vi "hse-configuration_ReadBooleanKey.vi"(8 "error in (no error)":errorcluster, 9 "Key":string, 10 "Section":string, 11 "hse-config-ini in":refnum<class "hse-config-ini.lvclass">) -> (0 "error out":errorcluster, 2 "Value":bool, 3 "hse-config-ini out":refnum<class "hse-config-ini.lvclass">)   [LabVIEW 2020, in "hse-config-ini.lvclass"]
doc: "Reads the numeric configuration value (I32) identified by <b>section</b> and <b>key</b> from the configuration object\n\n____\nHAMPEL SOFTWARE ENGINEERING v3.8.0 (2023-12-18 14:41)"
uses:
  hse-config-ini.lvclass
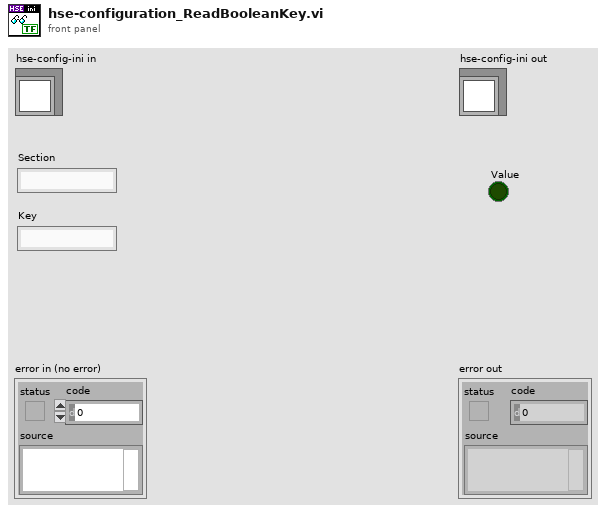
[diagram p1: front panel]
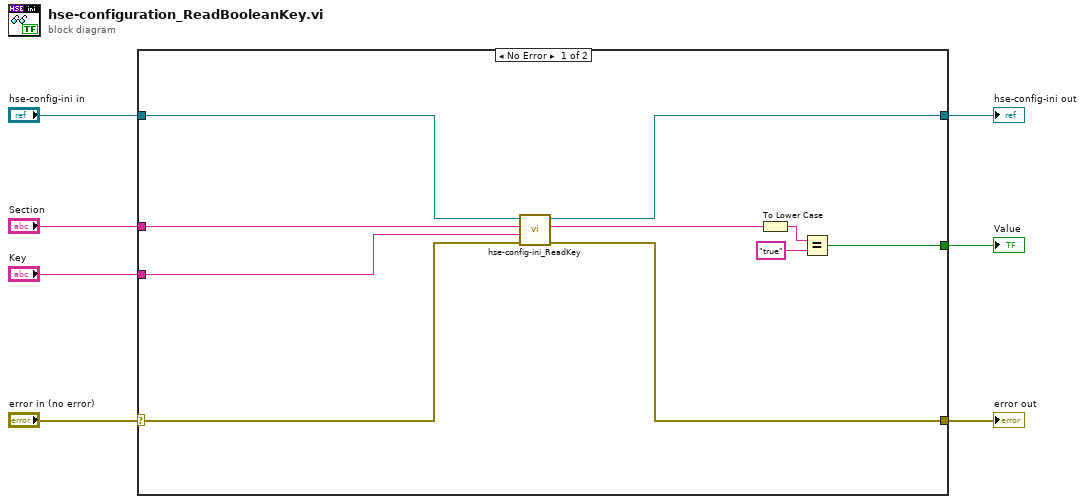
[diagram p0: block diagram]
diagram:
  n1 = case shown="No Error" "error in (no error)" {
    selector: "error in (no error)" -> [w13 w19]
    tunnel: [w12 w19] -> w7
    tunnel: "hse-config-ini in" -> [w17 w18]
    tunnel: [w16 w18] -> w4
    tunnel: "Section" -> [w15 _]
    tunnel: "Key" -> [w14 _]
    tunnel: [w10 _] -> w6
    frame No Error {
      n2 = call "hse-config-ini_ReadKey.vi"("error in (no error)"=w13, "Key"=w14, "Section"=w15, "hse-config-ini in"=w17) -> ("error out"=w12:errorcluster, "String"=w11:string, "hse-config-ini out"=w16:refnum<class "hse-config-ini.lvclass">)  [unwired: 5 in]
      n3 = To Lower Case(string=w11) -> (all lower case string=w8:string)
      n4 = Equal?(x=w8, y="true") -> (x = y?=w10:bool)
    }
    frame Error {
    }
  }
  "error out" <- w7
  "hse-config-ini out" <- w4
  "Value" <- w6
